vi "Convert Channel Values to Static Measure Digital Settings.vi"(9 "Length":i32, 10 "Index":i32, 11 "Channel Values in":dbl[](array[numeric])) -> (2 "Static Measure Digital Settings":T1, 3 "Channel Values out":dbl[](array[numeric]))   [LabVIEW 2018, in "FPGA Addon Engine.lvlib"]
uses:
  FPGA Addon Engine.lvlib
  Submodules/Source/Types/Static.Measure.Digital.Settings.ctl
  Submodules/Source/Speciality FPGA IO.lvlib
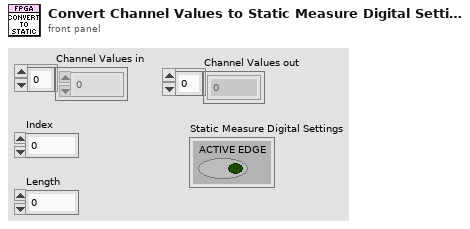
[diagram p1: front panel]
types:
  T1 = typedef "Speciality FPGA IO.lvlib/Static.Measure.Digital.Settings.ctl" = cluster{"ACTIVE EDGE":bool}
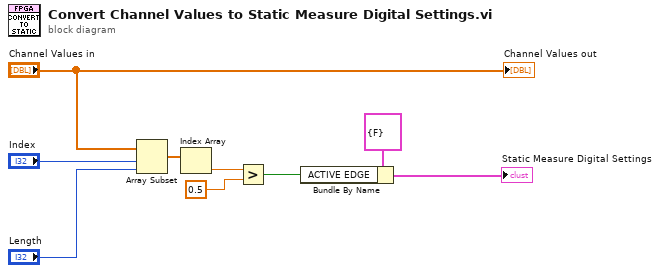
[diagram p0: block diagram]
diagram:
  n1 = Array Subset(array="Channel Values in", index="Index", length="Length") -> (w4:dbl[])
  n2 = Index Array(array=w4) -> (element=w1:dbl)  [unwired: 1 in]
  n3 = Greater?(x=w1, y=0.5) -> (0:w3:bool)
  n4 = Bundle By Name(cluster=T1 {"ACTIVE EDGE"=FALSE} ("Settings"), "ACTIVE EDGE"=w3) -> (→"Static Measure Digital Settings":T1)
  "Channel Values out" <- "Channel Values in"
